vi "Record_Initialization_2D.vi"(0 "Indexed Names":string[](array[string]), 1 "Refnum in":refnum<k34>, 2 "Period":i64, 3 "Buffer size":i64, 5 "Indexed SV Refnums":refnum<k21>[](array[refnum]), 7 "Indexed Type Code":i32[](array[numeric]), 11 "error in (no error)":errorcluster) -> (4 "2D Array of sizes":i32[][](array[numeric]), 6 "Array of channel names":string[][](array[string]), 8 "Array of 1D waveforms":waveform(dbl)[][](array[waveform]), 15 "error out":errorcluster)   [LabVIEW 2014]
doc: "<B>Copyright</B>: (c) MHWirth 2015. All rights are reserved.\n\nThis subVI sets the properties of the TDMS file for recording <B>2D arrays</B>, and prepares the name of channels for each group.\n\nEvery 2D array is saved in one group (sheet), and each element is saved in one channel (column)."
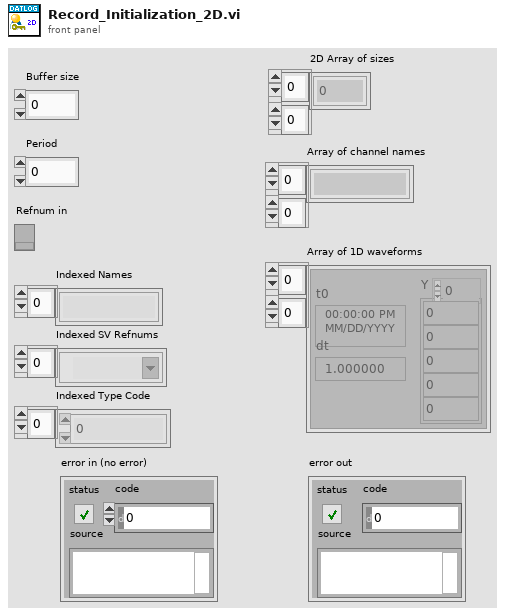
[diagram p1: front panel]
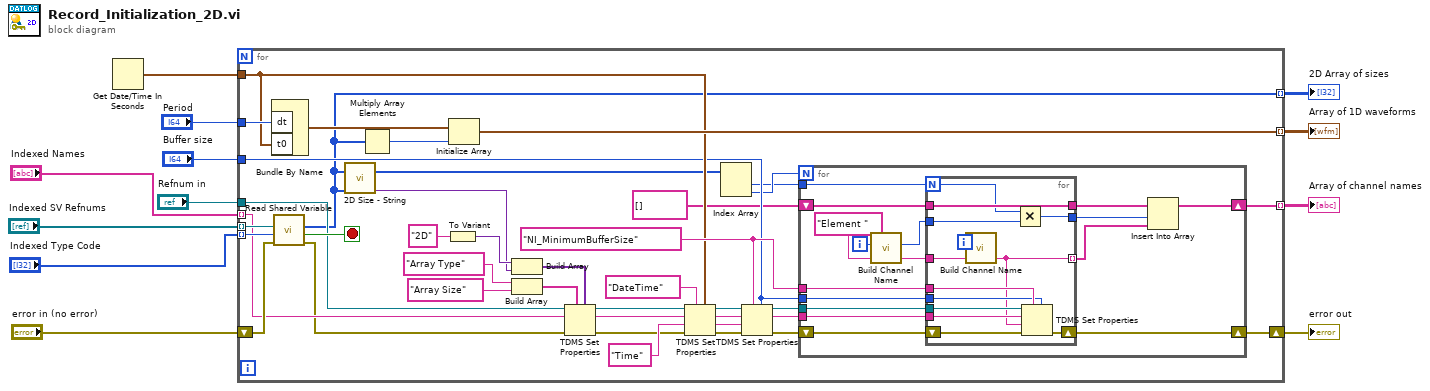
[diagram p0: block diagram]
diagram:
  n1 = Get Date/Time In Seconds() -> (seconds since 1Jan1904=w2:timestamp)
  n2 = for {
    tunnel: "Indexed Names" -> [w37] mode=indexing
    tunnel: "Indexed Type Code" -> [w49] mode=indexing
    tunnel: "Indexed SV Refnums" -> [w50] mode=indexing
    tunnel: "Refnum in" -> [w38]
    shift-right: [w25] -> w9
    shift-left: "error in (no error)" -> [w51]
    tunnel: "Buffer size" -> [w19]
    tunnel: [w14] -> w1 mode=indexing
    tunnel: w2 -> [w20]
    tunnel: "Period" -> [w32]
    tunnel: [w30] -> w12 mode=indexing
    tunnel: [w22] -> w11 mode=indexing
    stop <- w48 stop-if-true
    w21 = "NI_MinimumBufferSize"
    n3 = Bundle By Name("dt"=w32, "t0"=w20) -> (w31:waveform(dbl))  [unwired: 1 in]
    n4 = call "Read Shared Variable.vi"("Error In"=w51, "Type code"=w49, "Refnum"=w50) -> ("Error Out"=w36:errorcluster, "status"=w48:bool, "size(s)"=w14:i32[])  [unwired: 5 in, 1 out]
    n5 = call "2D Size - String.vi"("size(s)"=w14) -> ("size (string)"=w18:variant)  [unwired: 10 in]
    n6 = Multiply Array Elements(1:w14) -> (0:w17:i32)
    n7 = To Variant(anything="2D") -> (Variant=w34:variant)
    n8 = Initialize Array(w31, w17) -> (w30:waveform(dbl)[])
    n9 = Build Array(w34, w18) -> (w33:variant[])
    n10 = Build Array("Array Type", "Array Size") -> (w39:string[])
    n11 = TDMS Set Properties(5:w33, 7:w39, 8:w36, 10:w37, 11:w38) -> (0:w27:errorcluster, 2:w28:string, 3:w29:refnum<k34>)  [unwired: 1 in, 1 out]
    n12 = TDMS Set Properties(5:w20, 7:"DateTime" ("property names"), 8:w27, 9:"Time", 10:w28, 11:w29) -> (0:w47:errorcluster, 1:w46:string, 2:w45:string, 3:w44:refnum<k34>)
    n13 = Index Array(array=w14) -> (element #1=w15:i32, element #2=w16:i32)  [unwired: 2 in]
    n14 = TDMS Set Properties(5:w19, 7:w21, 8:w47, 9:w46, 10:w45, 11:w44) -> (0:w26:errorcluster, 2:w23:string, 3:w24:refnum<k34>)  [unwired: 1 out]
    n15 = for {
      N: w16 -> [_]
      shift-right: [w65] -> w25
      shift-left: w26 -> [w66]
      tunnel: w24 -> [w64]
      tunnel: w23 -> [w63]
      tunnel: w21 -> [w62]
      tunnel: w19 -> [w61]
      tunnel: w15 -> [w58]
      shift-right: [w57] -> w22
      shift-left: string[] [] -> [w54]
      i -> [w52]
      n16 = call "Build Channel Name.vi"("String in"="Element ", "Numeric"=w52) -> ("String out"=w59:string)  [unwired: 7 in]
      n17 = for {
        N: w58 -> [w68]
        tunnel: w64 -> [w77]
        tunnel: w63 -> [w76]
        tunnel: w62 -> [w75]
        tunnel: w61 -> [w74]
        shift-right: [w78] -> w65
        shift-left: w66 -> [w79]
        tunnel: w59 -> [w72]
        tunnel: [w71] -> w56 mode=indexing
        tunnel: [w70] -> w55
        tunnel: w54 -> [w70]
        tunnel: [w67] -> w53
        tunnel: w52 -> [w69]
        i -> [w73]
        n18 = call "Build Channel Name.vi"("String in"=w72, "Numeric"=w73) -> ("String out"=w71:string)  [unwired: 7 in]
        n19 = Multiply(x=w68, y=w69) -> (x*y=w67:i32)
        n20 = TDMS Set Properties(5:w74, 7:w75, 8:w79, 9:w71, 10:w76, 11:w77) -> (0:w78:errorcluster)  [unwired: 3 out]
      }
      n21 = Insert Into Array(array=w55, index=w53, new element=w56) -> (w57:string[])
    }
  }
  "Array of 1D waveforms" <- w12
  "Array of channel names" <- w11
  "error out" <- w9
  "2D Array of sizes" <- w1
